vi "APU 1.0 Read Outputs.vi"(5 "degrees of 1 crank u16":dbl, 7 "degrees of 1 cycle u16":dbl, 8 "error in (no error)":errorcluster, 9 "Device outputs in":dbl[](array[numeric]), 10 "output reference in":T1, 11 "FIFO indexes.outputs":T2) -> (0 "error out":errorcluster, 1 "Device outputs out":dbl[](array[numeric]), 2 "output reference out":T1)   [LabVIEW 2013, in "Engine Simulation Toolkit Engine.lvlib"]
uses:
  Engine Simulation Toolkit Engine.lvlib
  APU 1.0 Output Ref.ctl
  <vilib>/rvi/interface/common/niFpgaWaitOnOcc.vi
  <vilib>/Utility/error.llb/Error Cluster From Error Code.vi
  <vilib>/rvi/errors/niLvFpgaAdjustHostInterfaceError.vi
  <vilib>/rvi/interface/nirviReadWriteControl/nirviReadWriteControl.xnode
  NiFpgaLv.dll
  <vilib>/rvi/interface/Simulation/niFpgaSimulationCallBeginRW.vi
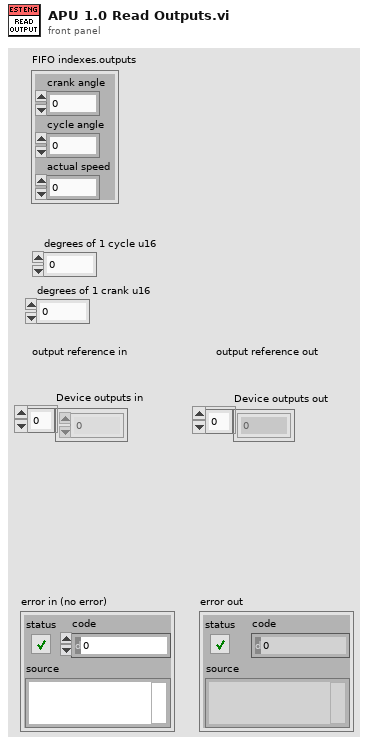
[diagram p1: front panel]
types:
  T1 = typedef "Engine Simulation Toolkit Engine.lvlib/APU 1.0 Output Ref.ctl" = refnum<k20>
  T2 = cluster{"crank angle":i32, "cycle angle":i32, "actual speed":i32}
  T3 = cluster{"crank":u16, "cycle":u16, "actual speed":fxp<+/-,23,2>}
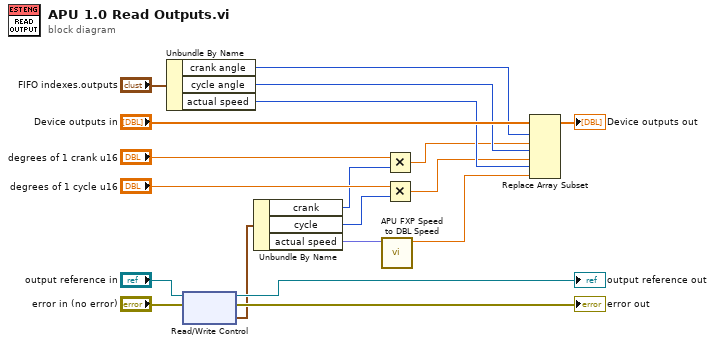
[diagram p0: block diagram]
diagram:
  n1 = Unbundle By Name("FIFO indexes.outputs") -> ("crank angle"=w12:i32, "cycle angle"=w11:i32, "actual speed"=w9:i32)
  n2 = xnode "Read/Write Control"("FPGA VI Reference In"="output reference in", "error in"="error in (no error)") -> ("FPGA VI Reference Out"=→"output reference out":T1, "error out"=→"error out":errorcluster, "Value"=w13:T3)
  n3 = Unbundle By Name(w13) -> ("crank"=w3:u16, "cycle"=w5:u16, "actual speed"=w8:fxp<+/-,23,2>)
  n4 = call "APU FXP Speed to DBL Speed.vi"("FXP speed"=w8) -> ("DBL speed"=w7:dbl)  [unwired: 10 in]
  n5 = Multiply(x="degrees of 1 crank u16", y=w3) -> (x*y=w1:dbl)
  n6 = Multiply(x="degrees of 1 cycle u16", y=w5) -> (x*y=w2:dbl)
  n7 = Replace Array Subset(array="Device outputs in", new element #1=w1, index #1=w12, new element #2=w2, index #2=w11, new element #3=w7, index #3=w9) -> (→"Device outputs out":dbl[])
